vi "dfd_Generate Bit Mask.vi"(11 "I32 max value":i32) -> (3 "U16 mask":u16 format="%.0x")   [LabVIEW 2017, in "NI_DigFilterLicensed.lvlib"]
uses:
  <vilib>/addons/Digital Filter Design/NI_DigFilterLicensed.lvlib
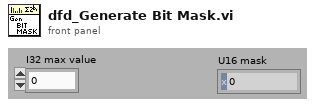
[diagram p1: front panel]
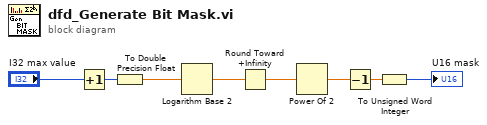
[diagram p0: block diagram]
diagram:
  n1 = Increment(x="I32 max value") -> (x+1=w1:i32)
  n2 = To Double Precision Float(number=w1) -> (double precision float=w8:dbl)
  n3 = Logarithm Base 2(1:w8) -> (0:w7:dbl)
  n4 = Round Toward +Infinity(x=w7) -> (ceil(x): smallest int >= x=w6:dbl)
  n5 = Power Of 2(x=w6) -> (2^x=w5:dbl)
  n6 = Decrement(x=w5) -> (x-1=w4:dbl)
  n7 = To Unsigned Word Integer(number=w4) -> (unsigned 16bit integer=→"U16 mask":u16)
